vi "List Categories.vi"(11 "Datastore.Dictionaries in":refnum<class "Datastore.Dictionaries.lvclass">) -> (1 "categories":string[](array[string]), 3 "Datastore.Dictionaries":refnum<class "Datastore.Dictionaries.lvclass">)   [LabVIEW 2021, in "Bananas.lvlib" / "Datastore.Dictionaries.lvclass"]
uses:
  Datastore.Dictionaries.lvclass
  Datastore.Dictionaries.lvclass/Datastore.Dictionaries.ctl
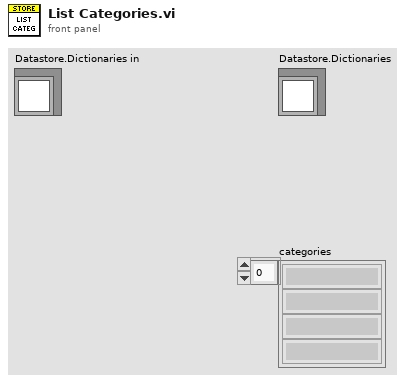
[diagram p1: front panel]
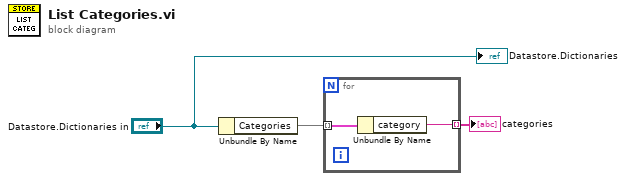
[diagram p0: block diagram]
diagram:
  n1 = Unbundle By Name("Datastore.Dictionaries in") -> ("Categories"=w3:map{string, map{string, variant}})
  n2 = for {
    tunnel: w3 -> [w5] mode=indexing
    tunnel: [w4] -> w2 mode=indexing
    n3 = Unbundle By Name(w5) -> ("category"=w4:string)
  }
  "categories" <- w2
  "Datastore.Dictionaries" <- "Datastore.Dictionaries in"
